vi "Get Provided Interface and Service Class.vi"(8 "error in":errorcluster, 11 "session factory in":refnum<class "KeysightDmm.lvclass">) -> (0 "error out":errorcluster, 1 "service class":string, 2 "provided interface":string, 3 "session factory out":refnum<class "KeysightDmm.lvclass">)   [LabVIEW 2021, in "KeysightDmm.lvclass"]
doc: "Returns the provided interface and service class that will be used to query the MeasurementLink Discovery Service for the address and port of the instrument's gRPC server. If your instrument does not use a gRPC server then you do not have to override this VI."
uses:
  KeysightDmm.lvclass
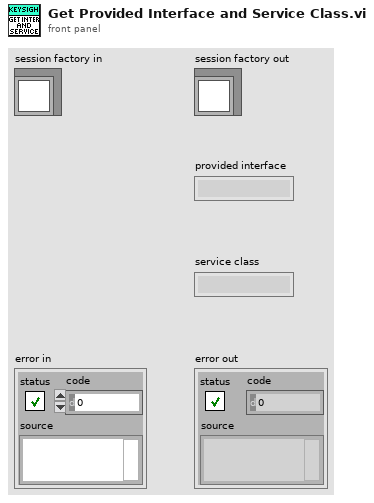
[diagram p1: front panel]
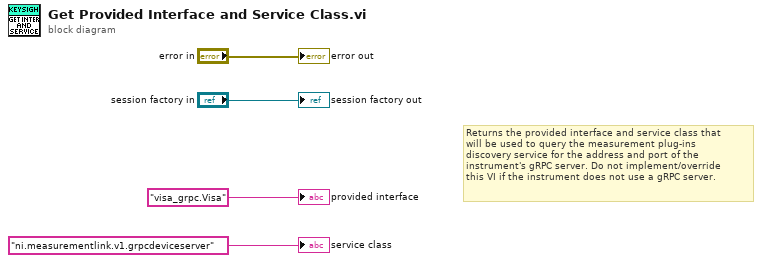
[diagram p0: block diagram]
diagram:
  # "Returns the provided interface and service class that \nwill be used to query the measurement plug-ins \ndiscovery service for the address and port of the \ninstrument's gRPC server. Do not implement/override \nthis VI if the instrument does not use a gRPC server."
  "error out" <- "error in"
  "session factory out" <- "session factory in"
  "provided interface" <- "visa_grpc.Visa" ("provided interface")
  "service class" <- "ni.measurementlink.v1.grpcdeviceserver" ("service class")
